vi "FGV_RunStatus.vi"(0 "Run Status":string, 4 "Enum":enum16{"Set", "Get"}(ring)) -> (5 "Run Status":string)   [LabVIEW 2018, in "feGEM DataPacker.lvlib"]
uses:
  feGEM DataPacker.lvlib
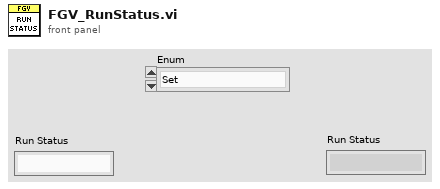
[diagram p1: front panel]
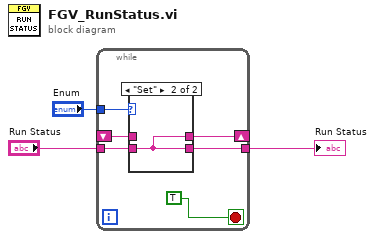
[diagram p0: block diagram]
diagram:
  n1 = while {
    shift-right: [w8] -> _
    shift-left: _ -> [w9]
    tunnel: "Run Status" -> [w6]
    tunnel: [w7] -> w2
    tunnel: "Enum" -> [w5]
    stop <- TRUE stop-if-true
    n2 = case shown="\"Set\"" w5 {
      tunnel: [w10 w11] -> w7
      tunnel: [w10 w11] -> w8
      tunnel: w9 -> [w10 _]
      tunnel: w6 -> [_ w11]
      frame "Get", Default {
      }
      frame "Set" {
      }
    }
  }
  "Run Status" <- w2
